vi "Is DataSocket.vi"(11 "String":string) -> (1 "After header":string, 2 "DataSocket":bool)   [LabVIEW 2021]
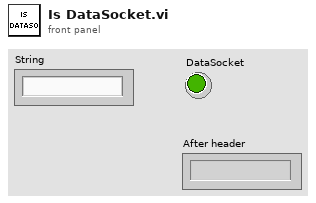
[diagram p1: front panel]
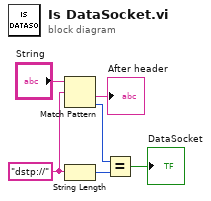
[diagram p0: block diagram]
diagram:
  w5 = "dstp://" ("regular expression")
  n1 = Match Pattern(string="String", regular expression=w5) -> (after substring=→"After header":string, offset past match=w6:i32)  [unwired: 1 in, 2 out]
  n2 = String Length(string=w5) -> (length=w4:i32)
  n3 = Equal?(x=w6, y=w4) -> (x = y?=→"DataSocket":bool)
